vi "Log Connect Event Helper.vi"(5 "Connecting":bool, 6 "Connected Argument":T1, 7 "State Info":string, 8 "error in (no error)":errorcluster, 9 "Arg:Connect":bool, 10 "STATUS.Connected":bool, 11 "EventLog in":refnum<class "EventLog.lvclass">) -> (0 "error out":errorcluster, 3 "EventLog out":refnum<class "EventLog.lvclass">)   [LabVIEW 2015, in "Tool Module.lvlib"]
uses:
  Tool Module.lvlib
  QC-X App/Libraries/Event Logger Library/Event Log/EventLog.lvclass
  Connected Argument--cluster.ctl
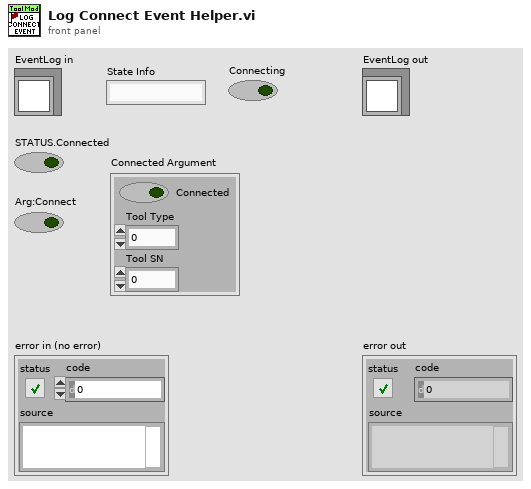
[diagram p1: front panel]
types:
  T1 = typedef "Tool Module.lvlib/Connected Argument--cluster.ctl" = cluster{"Connected":bool, "Tool Type":u16, "Tool SN":u16}
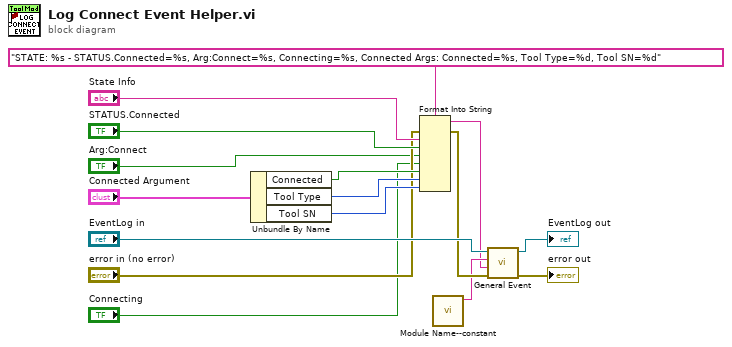
[diagram p0: block diagram]
diagram:
  n1 = Unbundle By Name("Connected Argument") -> ("Connected"=w8:bool, "Tool Type"=w7:u16, "Tool SN"=w6:u16)
  n2 = Format Into String(format string="STATE: %s - STATUS.Connected=%s, Arg:Connect=%s, Connecting=%s, Connected Args: Connected=%s, Tool Type=%d, Tool SN=%d", error in="error in (no error)", "State Info", "STATUS.Connected", "Arg:Connect", "Connecting", w8, w7, w6) -> (resulting string=w1:string, error out=w12:errorcluster)  [unwired: 1 in]
  n3 = call "Module Name--constant.vi"() -> ("Module Name"=w2:string)  [unwired: 11 in]
  n4 = call "General Event.vi"("error in (no error)"=w12, "Event Description"=w1, "Event Name"=w2, "EventLog ref"="EventLog in") -> ("error out"=→"error out":errorcluster, "EventLog ref"=→"EventLog out":refnum<class "EventLog.lvclass">)  [unwired: 6 in]
